vi "SENS_CORR_ISOL_STAT_ON_OFF_OBSOLETE.vi"(0 "VISA IN":refnum<visa-resource-name>, 1 "Isolation ON/OFF":bool, 5 "error in":errorcluster, 7 "Channel":i32) -> (14 "VISA Out":refnum<visa-resource-name>, 19 "error out":errorcluster)   [LabVIEW 2018, in "PNA-X.lvlib"]
doc: "SENSe<cnum>:CORRection:ISOLation[:STATe] <ON | OFF> OBSOLETE \nThis command no longer works beginning in the PNA 5.2 release. To perform isolation as part of an \nunguided calibration, you must explicitly measure the isolation standard using \nSENS:CORR:COLL:ACQ Stan5. See Example program. \nTo measure isolation as part of an ECal, use SENS:CORR:COLL:ISOL:ECAL. \n(Read-Write) Turns isolation cal ON or OFF during Full 2-port calibration. If this command is not \nsent, the default state is to disable Isolation. \nParameters \n<cnum> Any existing channel number. If unspecified, value is set to 1 \n<ON | OFF> ON (or 1) - turns isolation ON. \nOFF (or 0) - turns isolation OFF. \nExamples SENS:CORR:ISOL ON \nsense2:correction:isolation:state off \nQuery Syntax SENSe<cnum>:CORRection:ISOLation[:STATe]? \nReturn Type Boolean (1 = ON, 0 = OFF) \nDefault OFF - (Isolation disabled) \nSENSe:CORRection:PREFerence:CSET:SAVE <char> \n1632\n\nImportant Notes: \nThis command replaces SENS:CORR:PREF:CSET:SAVU \nWith 6.0 we implemented a change that defaults to saving completed calibrations to Cal Registers instead \nof User Cal Sets. To revert to the old behavior, send this command with the USER argument. \n(Read-Write) Specifies the default manner in which calibrations that are performed using SCPI or \nCOM are to be stored. Cal data is ALWAYS stored to the channel Cal Register regardless of this \nsetting. \nThis setting survives instrument preset and reboot. It remains until changed by another execution of \nthis command. \nNote: Cal Set arguments used with commands such as SENS:CORR:COLL:GUID:INIT, \nSENS:CORR:COLL:GUID:SAVE and SENS:CORR:COLL:GUID:SAVE:CSET will override of any \nof these default preference settings. \nLearn about Cal Registers and User Cal Sets. \nParameters \n<char> CALRegister - Cal is saved ONLY to the channel Cal Register. \nUSER - Cal is saved to a new User Cal Set file when performing a SCPI \ncalibration. The Cal Set name is automatically generated. To change the name, \nsend SENS:CORR:CSET:NAME after the cal is complete. This reverts to pre- \n6.0 behavior. \nREUSe - The cal is saved to the Cal Set that is currently selected on the \nspecified channel, which could be the channel Cal Register. If the channel does \nnot yet have a selected Cal Set, the cal will be saved to a new User Cal Set with \nan automatically-generated name. \nExamples SENS:CORR:PREF:CSET:SAVE USER \nsense:correction:preference:cset:save reuse \nQuery Syntax SENSe:CORRection:PREFerence:CSET:SAVE? \nReturn Type Character \nDefault CALRegister \nSENSe:CORRection:PREFerence:CSET:SAVUser <bool> Superseded \n1633\n\nThis command is replace with SENS:CORR:PREF:CSET:SAVE \nNOTE: With 6.0 we implemented a change that defaults to saving completed calibrations to Cal \nRegisters instead of User Cal Sets. To revert to the old behavior, send this command as ON (1). For \nUI and COM use, this can be done from the GPIB console. \n(Read-Write) Specifies whether cal data is automatically saved to a User Cal Set file after performing \na SCPI calibration. Cal data is always saved to a Cal Register regardless of this setting. \nThis setting survives instrument preset and reboot. It remains until changed by another execution of \nthis command. \nLearn about Cal Registers and User Cal Sets. \nParameters \n<bool> ON or 1 - Cal is automatically saved to a User Cal Set file when performing a \nSCPI calibration. The Cal Set name is automatically generated. To change the \nname, send SENS:CORR:CSET:NAME after the cal is complete. Reverts to \npre-6.0 behavior. \nOFF or 0 - Cal is NOT automatically saved to a User Cal Set. To save a \ncalibration to a User Cal Set, use SENS:CORR:COLL:GUID:INIT. \nExamples SENS:CORR:PREF:CSET:SAVU 1 \nsense:correction:preference:cset:savuser 0 \nQuery Syntax SENSe:CORRection:PREFerence:CSET:SAVUser? \nReturn Type Boolean (1 = ON, 0 = OFF) \nDefault OFF (0) \nSENSe:CORRection:PREFerence:ECAL:ORIentation[:STATe] <ON|OFF> \n1634\n\n(Read-Write) Specifies whether or not the PNA should perform orientation of the ECal module \nduring calibration. Orientation is a technique by which the PNA automatically determines which \nports of the module are connected to which ports of the PNA. Orientation begins to fail at very low \npower levels or if there is much attenuation in the path between the PNA and the ECal module. If \norientation is turned OFF, the SENS:CORR:PREF:ECAL:PMAP command must be used to specify \nthe port connections before performing a cal. \nNote: For 3-port or 4-port measurements, when orientation is OFF, you are not allowed to specify \nhow the ECAL module is connected. Instead, the PNA determines the orientation. Use \nSENS:CORR:COLL:GUID:DESC? to query the orientation. The PNA does not verify that you made \nthe connection properly. \nThis setting remains until the PNA is restarted or this command is sent again. \nParameters \n<bool> ECAL orientation state. Choose from: \nON or 1 - PNA performs orientation of the ECal module. \nOFF or 0 - PNA does NOT performs orientation of the ECal module. \nExamples SENS:CORR:PREF:ECAL:ORI OFF \nsense:correction:preference:ecal:orientation:state on \nQuery Syntax SENSe:CORRection:PREFerence:ECAL:ORIentation[:STATe]? \nReturn Type Boolean (1 = ON, 0 = OFF) \nDefault ON (1) \nSENSe:CORRection:PREFerence:ECAL:PMAP <module>,<string> \n(Read-Write) When ECal module orientation is turned OFF (SENS:CORR:PREF:ECAL:ORI), this \ncommand specifies the port mapping (which ports of the module are connected to which ports of the \nPNA) prior to performing ECal calibrations. \nThis setting remains until the PNA is restarted or this command is sent again. \nParameters \n<module> Specifies which ECal module this port map is being applied to. Choose from: \nECAL1 \n.through. \nECAL8 \n1635\n\n<string> Format this parameter in the following manner: \nAw,Bx,Cy,Dz \nwhere\nA, B, C, and D are literal ports on the ECAL module \nw,x,y, and z are substituted for PNA port numbers to which the ECAL module port \nis connected. \nPorts of the module which are not used are omitted from the string. \nFor example, on a 4-port ECal module with \nport A connected to PNA port 2 \nport B connected to PNA port 3 \nport C not connected \nport D connected to PNA port 1 \nthe string would be: A2,B3,D1 \nIf either the receive port or source port (or load port for 2-port cal) of the \nCALC:PAR:SELected measurement is not in this string and orientation is OFF, \nan attempt to perform an ECal calibration will fail. \nExamples SENS:CORR:PREF:ECAL:PMAP ECAL2, 'A1,B2' \nsense:correction:preference:ecal:pmap ecal3, 'a2,b1,c3' \nQuery Syntax SENSe:CORRection:PREFerence:ECAL:PMAP? <module> \nReturn Type String \nDefault Null string () \nSENSe:CORRection:PREFerence:SIMCal <bool> \n1636\n\n(Read-Write) Sets and returns a preference for the Unguided Cal behavior described below. This \nsetting persists until it is changed. \nThis preference can also be set True by executing the script on the PNA at C:/Program \nFiles/Agilent/Network Analyzer/System/wincal32.reg. \nParameters \n<bool> Boolean - Choose from: \n0 - False - Reverts to new (preferred) behavior. An error is returned if standard \ndata is not acquired before sending SENS:CORR:COLL:SAVE. \n1 - True - (WinCal compatible) Prevents SENS:CORR:COLL:SAVE from \nfailing when standard data has not, and will not, be acquired. \nLearn more about old and new behaviors. \nExamples SENS:CORR:PREF:SIMC 0 \nsense:correction:preference:simcal 1 \nQuery Syntax SENSe:CORRection:PREFerence:SIMCal? \nReturn Type Boolean \nDefault 0 \nSENSe:CORRection:PREFerence:TRIG:FREE <char>, <bool> \n(Read-Write) Sets and returns the preference for the trigger behavior during a calibration. This setting \npersists until it is changed. \nNote: If TRIGger:SOURce = Manual, during a calibration the PNA ALWAYS switches to Internal for \none trigger, then back to Manual, regardless of this preference command. \nParameters \n<char> Character - Calibration type. Choose from: \nGUIDed - preference setting pertains to a Guided calibration. \nUNGuided - preference setting pertains to an Unguided calibration. \n<bool> Boolean - Choose from: \n0 - False - The trigger behavior during the specified calibration type DOES \nrespect the setting of the TRIGger:SOURce command. For example,when \nTrigger source = External, the single trigger method will wait for the External \n1637\n\ntrigger signal and then allow only one sweep. \n1 - True - (Pre-6.0 behavior) The trigger behavior during the specified \ncalibration type does NOT respect the setting of the TRIGger:SOURce \ncommand. For example, when Trigger source = External, during calibration the \nPNA switches to Internal sweep, responds to one trigger signal to measure the \nstandard, then switches back to External. \nExamples SENS:CORR:PREF:TRIG:FREE GUID,1 \nsense:correction:preference:trig:free unguided,0 \nQuery Syntax SENSe:CORRection:PREFerence:TRIG:FREE? <char> \nReturn Type Boolean \nDefault False for both calibration types."
uses:
  PNA-X.lvlib
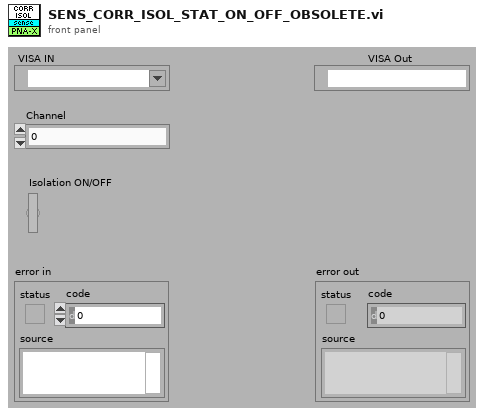
[diagram p1: front panel]
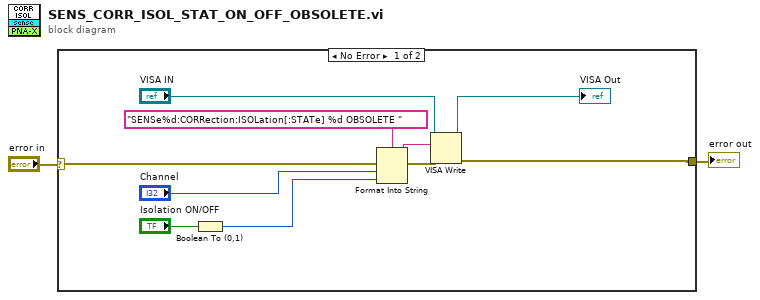
[diagram p0: block diagram]
diagram:
  n1 = case shown="No Error" "error in" {
    selector: "error in" -> [w12 w13]
    tunnel: [w7 w13] -> w1
    frame No Error {
      n2 = Boolean To (0,1)(Boolean="Isolation ON/OFF") -> (0, 1=w3:i16)
      n3 = Format Into String(format string="SENSe%d:CORRection:ISOLation[:STATe] %d OBSOLETE " ("Cmdline"), error in=w12, "Channel", w3) -> (resulting string=w10:string, error out=w11:errorcluster)  [unwired: 1 in]
      n4 = VISA Write(VISA resource name="VISA IN", write buffer=w10, error in (no error)=w11) -> (VISA resource name out=→"VISA Out":refnum<visa-resource-name>, error out=w7:errorcluster)  [unwired: 1 out]
    }
    frame Error {
    }
  }
  "error out" <- w1
